vi "Insert Scheduled Transfer Handles.vi"(4 "Label in":T1 {"Words"."Param Setting"."Num Bits" min=1 max=32; "Words"."Param Setting"."Start Bit" min=8 max=31; "Words"."Block Data Refs"."Data Reference" format="%.0x"; "Label" format="%.0o"}, 7 "Tx channel handle in":u32, 8 "error in (no error)":errorcluster) -> (0 "error out":errorcluster, 3 "Label out":T1 {"Words"."Param Setting"."Num Bits" min=1 max=32; "Words"."Param Setting"."Start Bit" min=8 max=31; "Words"."Block Data Refs"."Data Reference" format="%.0x"; "Label" format="%.0o"})   [LabVIEW 2012, in "AIT 429 Engine.lvlib"]
uses:
  RT Controls/RT Label Settings.ctl
  Shared/Controls and Global/Label.ctl
  Shared/Controls and Global/transferPeriod.ctl
  RT Controls/Driver Data.ctl
  RT Controls/RT Word Settings.ctl
  <vilib>/NI Veristand/Custom Device API/Block Data Reference.ctl
  <vilib>/NI Veristand/Custom Device API/Data Reference.ctl
  RT Controls/RT Param Setting.ctl
  Shared/Controls and Global/Start Bit.ctl
  Shared/Controls and Global/Number of Bits.ctl
  Shared/Controls and Global/TransferType.ctl
  AIT 429 Engine.lvlib
  <instrlib>/AIT 429/AIT 429.lvlib
  ARINC 429 Shared.lvlib
  <vilib>/NI Veristand/Custom Device API/Custom Device API.lvlib
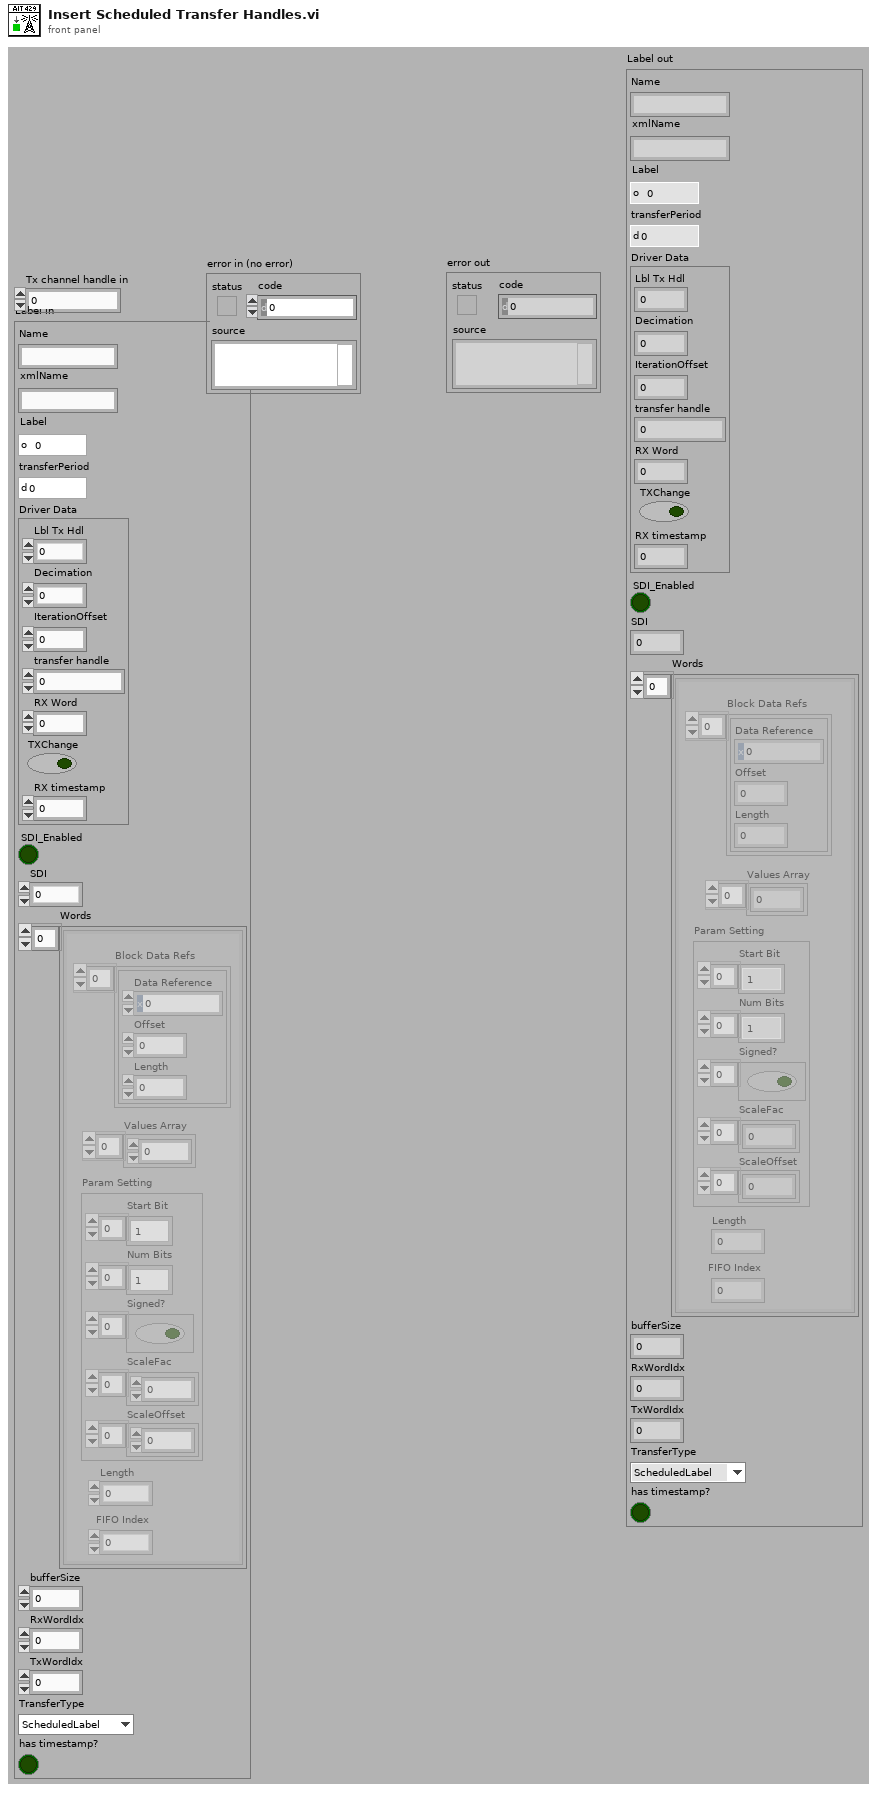
[diagram p1: front panel]
types:
  T1 = typedef "AIT 429 Engine.lvlib/RT Label Settings.ctl" = cluster{"Name":string, "xmlName":string, "Label":T2, "transferPeriod":T3, "Driver Data":T4, "SDI_Enabled":bool, "SDI":u8, "Words":T5[], "bufferSize":u32, "RxWordIdx":i32, "TxWordIdx":i32, "TransferType":T11, "has timestamp?":bool}
  T2 = typedef "ARINC 429 Shared.lvlib/Label.ctl" = u8
  T3 = typedef "ARINC 429 Shared.lvlib/transferPeriod.ctl" = u32
  T4 = typedef "AIT 429 Engine.lvlib/Driver Data.ctl" = cluster{"Lbl Tx Hdl":u32, "Decimation":i32, "IterationOffset":i32, "transfer handle":u32, "RX Word":u32, "TXChange":bool, "RX timestamp":dbl}
  T5 = typedef "AIT 429 Engine.lvlib/RT Word Settings.ctl" = cluster{"Block Data Refs":T6[], "Values Array":dbl[], "Length":i32, "FIFO Index":i32, "Param Setting":T8}
  T6 = typedef "Custom Device API.lvlib/Block Data Reference.ctl" = cluster{"Data Reference":T7, "Offset":i32, "Length":i32}
  T7 = typedef "Custom Device API.lvlib/Data Reference.ctl" = i32
  T8 = typedef "AIT 429 Engine.lvlib/RT Param Setting.ctl" = cluster{"Start Bit":T9[], "Num Bits":T10[], "Signed?":bool[], "ScaleFac":dbl[], "ScaleOffset":dbl[]}
  T9 = typedef "ARINC 429 Shared.lvlib/Start Bit.ctl" = i32
  T10 = typedef "ARINC 429 Shared.lvlib/Number of Bits.ctl" = i32
  T11 = typedef "ARINC 429 Shared.lvlib/TransferType.ctl" = enum16{"ScheduledLabel", "Acyclic", "Block", "Strobe"}
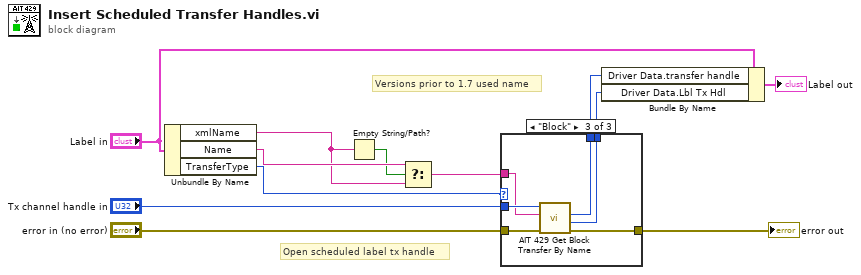
[diagram p0: block diagram]
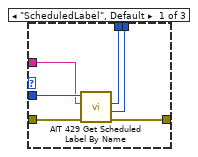
[diagram p2: hidden frame]
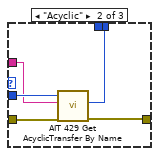
[diagram p3: hidden frame]
diagram:
  # "Open scheduled label tx handle"
  # "Versions prior to 1.7 used name"
  n1 = Unbundle By Name("Label in") -> ("xmlName"=w5:string, "Name"=w6:string, "TransferType"=w1:T11)
  n2 = Empty String/Path?(string/path=w5) -> (empty?=w3:bool)
  n3 = Select(t=w6, s=w3, f=w5) -> (s? t:f=w2:string)
  n4 = case shown="\"Block\"" w1 {
    tunnel: "error in (no error)" -> [w18 w23 w29]
    tunnel: [w17 w19 w25] -> w9
    tunnel: [w16 _ w26] -> w8
    tunnel: "Tx channel handle in" -> [w15 w21 w27]
    tunnel: [w14 w22 w28] -> w4
    tunnel: w2 -> [w13 w20 w24]
    frame "ScheduledLabel", Default {
      n5 = call <instrlib>:"AIT 429 Get Scheduled Label By Name.vi"("error in"=w18, "transfer name"=w13, "Tx channel handle in"=w15) -> ("error out"=w14:errorcluster, "scheduled label transfer handle out"=w17:u32, "rate oriented transfer handle out"=w16:u32)  [unwired: 3 in, 1 out]
    }
    frame "Acyclic" {
      n6 = call <instrlib>:"AIT 429 Get AcyclicTransfer By Name.vi"("error in"=w23, "transfer name"=w20, "channel handle"=w21) -> ("error out"=w22:errorcluster, "acyclic transfer handle out"=w19:u32)  [unwired: 6 in, 1 out]
    }
    frame "Block" {
      n7 = call <instrlib>:"AIT 429 Get Block Transfer By Name.vi"("error in"=w29, "transfer name"=w24, "Tx channel handle in"=w27) -> ("error out"=w28:errorcluster, "block transfer handle out"=w25:u32, "rate oriented transfer handle out"=w26:u32)  [unwired: 3 in, 1 out]
    }
  }
  "error out" <- w4
  n8 = Bundle By Name(cluster="Label in", "Driver Data.transfer handle"=w8, "Driver Data.Lbl Tx Hdl"=w9) -> (→"Label out":T1)
